vi "testing_delay_pair_sweep.vi"() -> ()   [LabVIEW 2015, in "Tausand AB1000.lvlib"]
uses:
  <instrlib>/Tausand AB1000/Tausand AB1000.lvlib
  <instrlib>/Tausand AB1000/Public/Controls/deviceTypeRing.ctl
  <instrlib>/Tausand AB1000/Public/Controls/channelRing.ctl
panel:
  out "combined graph":cluster{i32[], i32[]}[](graph)
  out "delay ch2":u32 caption="delay B"
  out "delay ch1":u32 caption="delay A"
  out "data array":i32[][](array[numeric])
  out "cc graph":cluster{i32[], i32[]}(graph)
  out "c2 graph":cluster{i32[], i32[]}(graph)
  out "c1 graph":cluster{i32[], i32[]}(graph)
  in  "delayed channel 2":T1=2 items=["none", "A", "B", "C", "D", "E", "F", "G", "H"]
  in  "delayed channel 1":T1=1 items=["none", "A", "B", "C", "D", "E", "F", "G", "H"]
  in  "cw (ns)":u32=10
  out "i case":i32
  out "total cases":i32
  in  "Stop Button":bool
  in  "sampling (ms)":u32=1000
  out "i delay":i32
  out "device type":T2 items=["any"=0, "AB1002"=1002, "AB1004"=1004, "AB1502"=1502, "AB1504"=1504, "AB1902"=1902, "AB1904"=1904]
  out "delay array":i32[](array[numeric])
  in  "step delay (ns)":i32=1
  in  "max delay (ns)":u32=20
  out "current delay (ns)":i32
  in  "VISA resource name":refnum<visa-resource-name>
  # "case"
  # "out of"
  # "Delay (ns)    counts 1      counts 2      coincid."
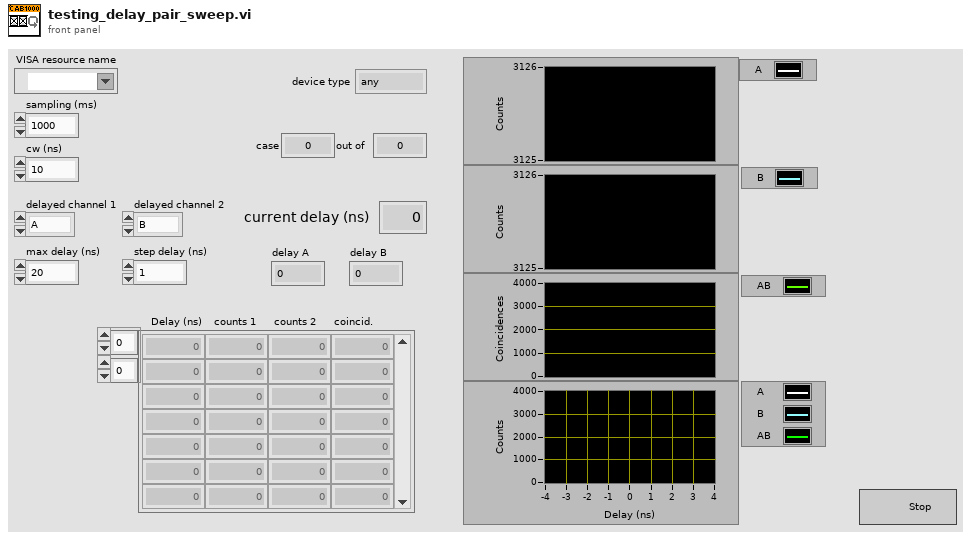
[diagram p1: front panel]
types:
  T1 = typedef "Tausand AB1000.lvlib/channelRing.ctl" = u8
  T2 = typedef "Tausand AB1000.lvlib/deviceTypeRing.ctl" = u16
  T3 = typedef "Tausand AB1000.lvlib/counters4ch.ctl" = cluster{"counter_A":u32, "counter_B":u32, "counter_C":u32, "counter_D":u32, "counter_AB":u32, "counter_AC":u32, "counter_AD":u32, "counter_BC":u32, "counter_BD":u32, "counter_CD":u32, "counter_multiple_1":u32, "counters_ID":u32, "time_left":u32}
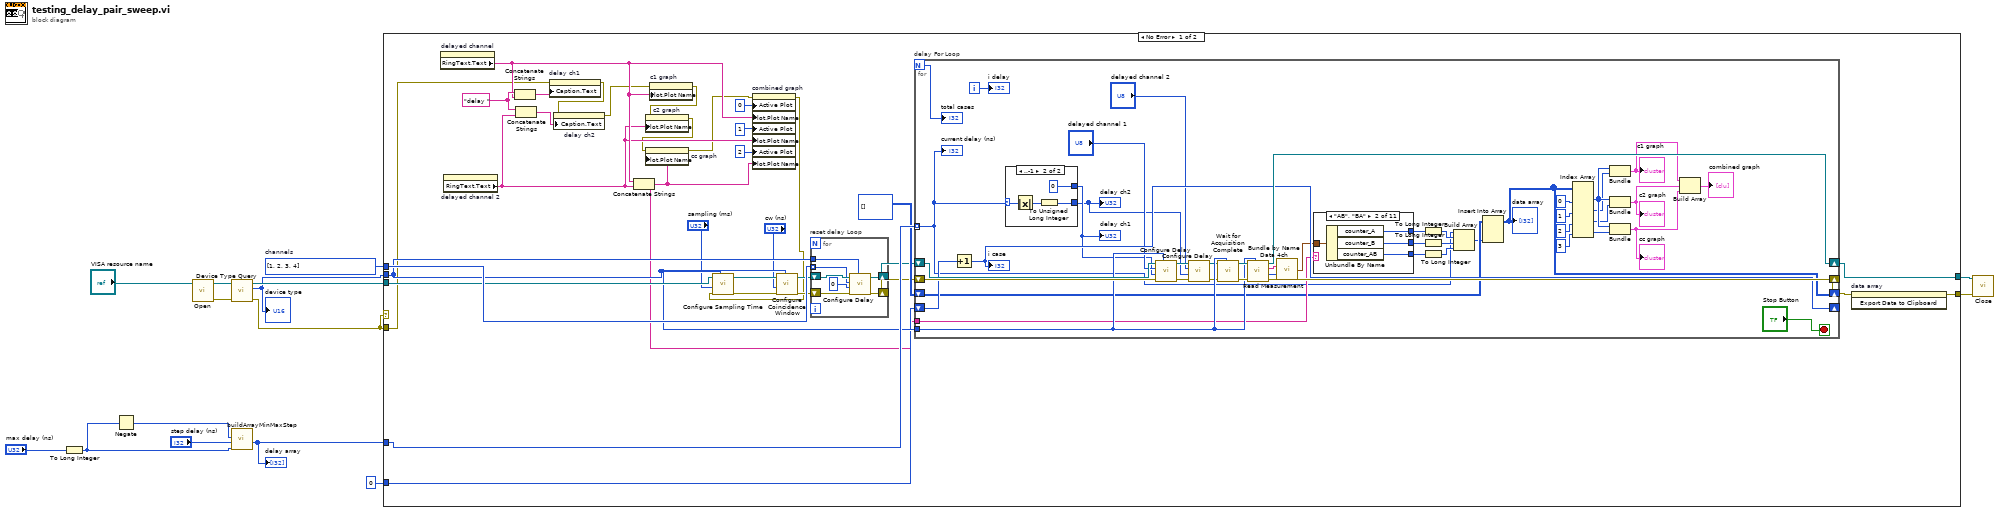
[diagram p0: block diagram]
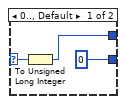
[diagram p2: hidden frame]
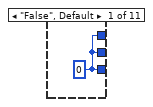
[diagram p3: hidden frame]
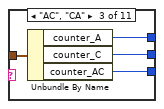
[diagram p4: hidden frame]
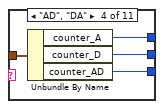
[diagram p5: hidden frame]
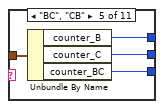
[diagram p6: hidden frame]
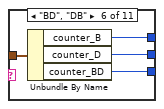
[diagram p7: hidden frame]
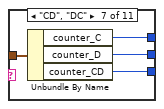
[diagram p8: hidden frame]
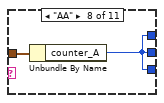
[diagram p9: hidden frame]
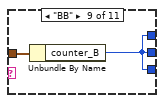
[diagram p10: hidden frame]
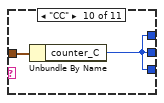
[diagram p11: hidden frame]
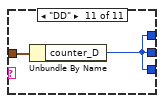
[diagram p12: hidden frame]
diagram:
  w8 = T1[] [1, 2, 3, 4] items=["none", "A", "B", "C", "D", "E", "F", "G", "H"]  # channels
  n1 = To Long Integer(number="max delay (ns)") -> (32bit integer=w1:i32)
  n2 = Negate(x=w1) -> (-x=w3:i32)
  n3 = call <instrlib>:"Open.vi"("VISA resource name"="VISA resource name") -> ("error out"=w13:errorcluster, "VISA resource name out"=w12:refnum<visa-resource-name>)  [unwired: 9 in]
  n4 = call <instrlib>:"Device Type Query.vi"("error in (no error)"=w13, "VISA Refnum in"=w12) -> ("error out"=w5:errorcluster, "device type"=w10:T2, "VISA Refnum out"=w11:refnum<visa-resource-name>)  [unwired: 7 in]
  "device type" <- w10
  n5 = call <instrlib>:"buildArrayMinMaxStep.vi"("max (10)"=w1, "step (1)"="step delay (ns)", "min (0)"=w3) -> ("array"=w9:i32[])  [unwired: 8 in]
  "delay array" <- w9
  n6 = case shown="No Error" w5 {
    tunnel: w5 -> [w17 w143]
    tunnel: w11 -> [w45 w142]
    tunnel: w10 -> [w44 _]
    tunnel: w9 -> [w48 _]
    tunnel: w8 -> [w46 _]
    tunnel: [w47 w142] -> w7
    tunnel: [w32 w143] -> w6
    tunnel: 0 ("i delay") -> [w40 _]
    frame No Error {
      w30 = "delay "
      n7 = property on="delayed channel" class="Ring (strict)"() -> ("RingText.Text"=w25:string)  [unwired: 2 in, 2 out]
      n8 = property on="delayed channel 2" class="Ring (strict)"() -> ("RingText.Text"=w24:string)  [unwired: 2 in, 2 out]
      n9 = Concatenate Strings(w30, w25) -> (w31:string)
      n10 = Concatenate Strings(w30, w24) -> (w29:string)
      n11 = property on="delay ch1" class="DigNum (strict)"(error in=w17, "Caption.Text"=w31) -> (error out=w19:errorcluster)  [unwired: 1 in, 1 out]
      n12 = property on="delay ch2" class="DigNum (strict)"(error in=w19, "Caption.Text"=w29) -> (error out=w18:errorcluster)  [unwired: 1 in, 1 out]
      n13 = Concatenate Strings(w25, w24) -> (w23:string)
      n14 = property on="c1 graph" class="XYGraph (strict)"(error in=w18, "Plot.Plot Name"=w25) -> (error out=w22:errorcluster)  [unwired: 1 in, 1 out]
      n15 = property on="c2 graph" class="XYGraph (strict)"(error in=w22, "Plot.Plot Name"=w24) -> (error out=w21:errorcluster)  [unwired: 1 in, 1 out]
      n16 = property on="cc graph" class="XYGraph (strict)"(error in=w21, "Plot.Plot Name"=w23) -> (error out=w20:errorcluster)  [unwired: 1 in, 1 out]
      n17 = property on="combined graph" class="XYGraph (strict)"(error in=w20, "Active Plot"=u32 0, "Plot.Plot Name"=w25, "Active Plot"=u32 1, "Plot.Plot Name"=w24, "Active Plot"=u32 2, "Plot.Plot Name"=w23) -> (error out=w16:errorcluster)  [unwired: 1 in, 1 out]
      n18 = call <instrlib>:"Configure Sampling Time.vi"("device type"=w44, "error in (no error)"=w16, "value (1000 ms)"="sampling (ms)", "VISA Refnum in"=w45) -> ("error out"=w42:errorcluster, "VISA Refnum out"=w41:refnum<visa-resource-name>)  [unwired: 5 in, 1 out]
      n19 = call <instrlib>:"Configure Coincidence Window.vi"("device type"=w44, "error in (no error)"=w42, "value ns (10ns)"="cw (ns)", "VISA Refnum in"=w41) -> ("error out"=w38:errorcluster, "VISA Refnum out"=w39:refnum<visa-resource-name>)  [unwired: 5 in, 1 out]
      n20 = for "reset delay Loop" {
        tunnel: w46 -> [w54] mode=indexing
        tunnel: w44 -> [w52]
        shift-right: [w50] -> w34
        shift-left: w38 -> [w51]
        shift-right: [w49] -> w35
        shift-left: w39 -> [w55]
        n21 = call <instrlib>:"Configure Delay.vi"("device type"=w52, "error in (no error)"=w51, "value (0 ns)"=u32 0, "channel"=w54, "VISA Refnum in"=w55) -> ("error out"=w50:errorcluster, "VISA Refnum out"=w49:refnum<visa-resource-name>)  [unwired: 4 in, 1 out]
      }
      n22 = for "delay For Loop" {
        N -> [w88]
        tunnel: w48 -> [w62] mode=indexing
        tunnel: w44 -> [w95]
        shift-right: [w99] -> w33
        shift-left: w34 -> [w100]
        shift-right: [w98] -> w47
        shift-left: w35 -> [w101]
        shift-right: [w89] -> _
        shift-left: w40 -> [w90]
        tunnel: w23 -> [w87]
        shift-right: [w79] -> _
        shift-left: i32[][] [] -> [w85]
        i -> [w91]
        stop <- "Stop Button" stop-if-true
        n23 = Increment(x=w90) -> (x+1=w89:i32)
        "i case" <- w89
        n24 = case shown="..-1" w62 {
          selector: w62 -> [w104 w108]
          tunnel: [w102 u32 0] -> w61
          tunnel: [u32 0 w105] -> w60
          frame 0.., Default {
            n25 = To Unsigned Long Integer(number=w104) -> (unsigned 32bit integer=w102:u32)
          }
          frame ..-1 {
            n26 = Absolute Value(x=w108) -> (abs(x)=w107:i32)
            n27 = To Unsigned Long Integer(number=w107) -> (unsigned 32bit integer=w105:u32)
          }
        }
        "delay ch1" <- w61
        "delay ch2" <- w60
        n28 = call <instrlib>:"Configure Delay.vi"("device type"=w95, "error in (no error)"=w100, "value (0 ns)"=w61, "channel"="delayed channel 1", "VISA Refnum in"=w101) -> ("error out"=w68:errorcluster, "VISA Refnum out"=w66:refnum<visa-resource-name>)  [unwired: 4 in, 1 out]
        n29 = call <instrlib>:"Configure Delay.vi"("error in (no error)"=w68, "value (0 ns)"=w60, "channel"="delayed channel 2", "VISA Refnum in"=w66) -> ("error out"=w67:errorcluster, "VISA Refnum out"=w65:refnum<visa-resource-name>)  [unwired: 5 in, 1 out]
        n30 = call <instrlib>:"Wait for Acquisition Complete.vi"("device type"=w95, "error in (no error)"=w67, "VISA resource name"=w65) -> ("error out"=w97:errorcluster, "VISA resource name out"=w96:refnum<visa-resource-name>)  [unwired: 7 in]
        n31 = call <instrlib>:"Read Measurement.vi"("device type"=w95, "error in (no error)"=w97, "VISA Refnum in"=w96) -> ("error out"=w99:errorcluster, "values"=w93:u32[], "labels"=w94:string[], "VISA Refnum out"=w98:refnum<visa-resource-name>)  [unwired: 3 in, 2 out]
        n32 = call <instrlib>:"Bundle by Name Data 4ch.vi"("names"=w94, "values"=w93) -> ("output cluster 4ch"=w86:T3)  [unwired: 13 in]
        n33 = case shown="\"AB\", \"BA\"" w87 {
          tunnel: w86 -> [_ w113 w117 w121 w125 w129 w133 w135 w137 w139 w141]
          tunnel: [w109 w112 w116 w120 w124 w128 w132 w134 w136 w138 w140] -> w81
          tunnel: [w109 w111 w115 w119 w123 w127 w131 w134 w136 w138 w140] -> w70
          tunnel: [w109 w110 w114 w118 w122 w126 w130 w134 w136 w138 w140] -> w69
          frame "False", Default {
            w109 = u32 0 ("counter_AB")
          }
          frame "AB", "BA" {
            n34 = Unbundle By Name(w113) -> ("counter_A"=w111:u32, "counter_B"=w110:u32, "counter_AB"=w112:u32)
          }
          frame "AC", "CA" {
            n35 = Unbundle By Name(w117) -> ("counter_A"=w115:u32, "counter_C"=w114:u32, "counter_AC"=w116:u32)
          }
          frame "AD", "DA" {
            n36 = Unbundle By Name(w121) -> ("counter_A"=w119:u32, "counter_D"=w118:u32, "counter_AD"=w120:u32)
          }
          frame "BC", "CB" {
            n37 = Unbundle By Name(w125) -> ("counter_B"=w123:u32, "counter_C"=w122:u32, "counter_BC"=w124:u32)
          }
          frame "BD", "DB" {
            n38 = Unbundle By Name(w129) -> ("counter_B"=w127:u32, "counter_D"=w126:u32, "counter_BD"=w128:u32)
          }
          frame "CD", "DC" {
            n39 = Unbundle By Name(w133) -> ("counter_C"=w131:u32, "counter_D"=w130:u32, "counter_CD"=w132:u32)
          }
          frame "AA" {
            n40 = Unbundle By Name(w135) -> ("counter_A"=w134:u32)
          }
          frame "BB" {
            n41 = Unbundle By Name(w137) -> ("counter_B"=w136:u32)
          }
          frame "CC" {
            n42 = Unbundle By Name(w139) -> ("counter_C"=w138:u32)
          }
          frame "DD" {
            n43 = Unbundle By Name(w141) -> ("counter_D"=w140:u32)
          }
        }
        n44 = To Long Integer(number=w70) -> (32bit integer=w83:i32)
        n45 = To Long Integer(number=w69) -> (32bit integer=w82:i32)
        n46 = To Long Integer(number=w81) -> (32bit integer=w80:i32)
        n47 = Build Array(w62, w83, w82, w80) -> (w84:i32[])
        n48 = Insert Into Array(array=w85, new element=w84) -> (w79:i32[][])  [unwired: 2 in]
        "data array" <- w79
        n49 = Index Array(array=w79, index (col) #1=0 ("disabled index (col)"), index (col) #2=1 ("index (col)"), index (col) #3=2 ("index (col)"), index (col) #4=3 ("index (col)")) -> (element #1=w74:i32[], element #2=w73:i32[], element #3=w72:i32[], element #4=w71:i32[])  [unwired: 4 in]
        n50 = Bundle(w74, w73) -> (w59:cluster{i32[], i32[]})  [unwired: 1 in]
        "c1 graph" <- w59
        n51 = Bundle(w74, w72) -> (w58:cluster{i32[], i32[]})  [unwired: 1 in]
        "c2 graph" <- w58
        n52 = Bundle(w74, w71) -> (w57:cluster{i32[], i32[]})  [unwired: 1 in]
        "cc graph" <- w57
        n53 = Build Array(w59, w58, w57) -> (→"combined graph":cluster{i32[], i32[]}[])
        "i delay" <- w91
        "total cases" <- w88
        "current delay (ns)" <- w62
      }
      n54 = invoke on="data array" class="Arr (strict)" method="Export Data to Clipboard"(error in=w33) -> (error out=w32:errorcluster)  [unwired: 2 in, 2 out]
    }
    frame Error {
    }
  }
  n55 = call <instrlib>:"Close.vi"("error in (no error)"=w6, "VISA resource name"=w7) -> ()  [unwired: 9 in, 1 out]
